vi "Write_Data.vi"(8 "error in (no error)":errorcluster caption="entrée d'erreur (pas d'erreur)", 10 "Data_To_Write":string, 11 "Class Instrument Power_Supply en entrée":refnum<class "Class Instrument Power_Supply.lvclass">) -> (0 "error out":errorcluster caption="sortie d'erreur", 3 "Class Instrument Power_Supply en sortie":refnum<class "Class Instrument Power_Supply.lvclass">)   [LabVIEW 2020, in "Library Instrument & Equipement.lvlib" / "Library Instruments.lvlib" / "Class Instrument Power_Supply.lvclass"]
uses:
  Class Instrument Power_Supply.lvclass
  Commun VI/TypeDef/Command Power_Supply/Data_Write_Power_Supply.ctl
  JSON API/JSON Value/Set from JSON string.vi
  JSON API/JSON Value/JSON Value.lvclass
  Class Instrument Power_Supply.lvclass/Class Instrument Power_Supply.ctl
  Commun VI/Library Commun.lvlib
  JSON API/Variant JSON/Variant JSON.lvlib
  JSON API/Get Polymorphic/JSON GetSet.lvlib
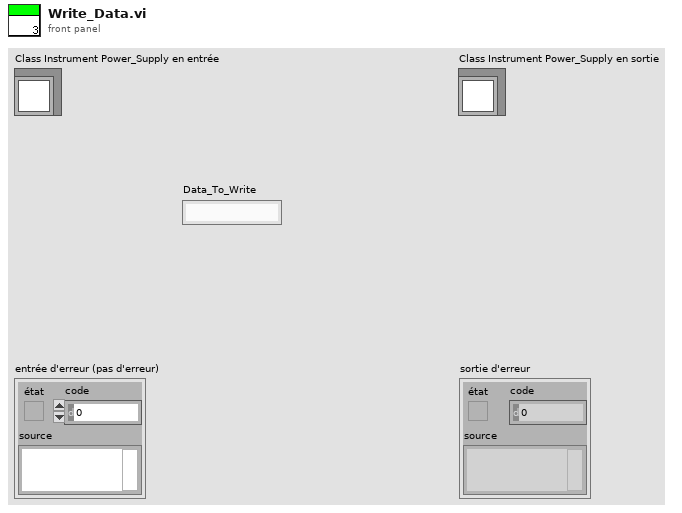
[diagram p1: front panel]
types:
  T1 = typedef "Library Commun.lvlib/Data_Write_Power_Supply.ctl" = enum16{"Enable Channel", "Disable Channel"}
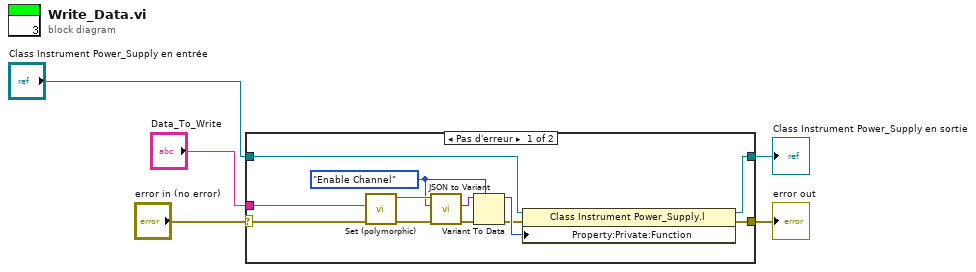
[diagram p0: block diagram]
diagram:
  n1 = case shown="Pas d'erreur" "error in (no error)" {
    selector: "error in (no error)" -> [w7 w19]
    tunnel: [w16 w19] -> w4
    tunnel: [w15 w18] -> w2
    tunnel: "Class Instrument Power_Supply en entrée" -> [w17 w18]
    tunnel: "Data_To_Write" -> [w9 _]
    frame No Error {
      w10 = Data_Write_Power_Supply."Enable Channel" ("Function")
      n2 = call-poly "Set (polymorphic).vi"("error in (no error)"=w7, "JSON stream"=w9) -> ("error out"=w13:errorcluster, "JSON Value out"=w11:refnum<class "JSON Value.lvclass">)  [unwired: 7 in, 1 out]
      n3 = call "JSON to Variant.vi"("error in (no error)"=w13, "Variant (Data Type)"=w10, "JSON Value"=w11) -> ("error out"=w12:errorcluster, "Variant out"=w14:variant)  [unwired: 7 in]
      n4 = Variant To Data(error in=w12, type=w10, Variant=w14) -> (data=w8:T1, error out=w6:errorcluster)
      n5 = property class="Class Instrument Power_Supply.l"(reference=w17, error in=w6, "Property:Private:Function"=w8) -> (reference out=w15:refnum<class "Class Instrument Power_Supply.lvclass">, error out=w16:errorcluster)
    }
    frame Error {
    }
  }
  "error out" <- w4
  "Class Instrument Power_Supply en sortie" <- w2
